vi "EnFlo_Tunnel_Display.vi"(4 "End Time":dbl, 5 "Start Time":dbl, 6 "Channel Values":dbl[](array[numeric]) format="%.3f", 7 "Ch names":string[](array[string])) -> ()   [LabVIEW 2016]
uses:
  Anemometry Sub Vis/Data_plotting_vis/File_Template_Clus.ctl
  Anemometry Sub Vis/Controls/Global_mode.ctl
  Anemometry Sub Vis/Globals/Constants_global.vi
  Anemometry Sub Vis/Data_plotting_vis/Results_plotter_Global.vi
  <vilib>/gmath/NI_Gmath.lvlib
panel:
  out "Inlet Door Heater Power %":dbl format="%#.2g"
  out "Exit Heater Power %":dbl format="%#.2g"
  out "Averaging time (minutes)":dbl format="%#.1f"
  out "End time":timestamp format="%<%H:%M\n%x>T"
  out "Start time":timestamp format="%<%H:%M\n%x>T"
  out "Top Level":bool
  out "Loop number":i32
  out "Lateral profiles":cluster{"Y Axis Current":dbl[], dbl[]}[](graph)
  out "Setpoints":dbl[](array[numeric])
  in  "Subtract Setpoint?":bool
  out "Vert Disp (mm)  @ 14m":dbl
  out "Inlet St Dev":dbl format="%#.3g"
  out "Inlet mapping":dbl[][](graph)=[[0.00729, 0.18153463174730816, 0.17352738437348433, 1.6752433719500537, 8.231465735195274, 17.570357598383207, 23.099772817121426, 25.58386930448374, 25.31727725753219, 24.28926231541072, 18.717383219374323, 10.355253339797807, 2.7760273383248344, 0.3109897541921306, 0.08276881403435009, 0.06197], [0.04411, 0.1361526368018142, 0.04039202183336771, 1.5611636795339547, 8.176972694107874, 17.32000974741714, 24.257541358764026, 25.949153465972987, 26.01802540761648, 25.060373307424115, 18.284750328365213, 8.689831176707928, 2.642937641487066, 0.43219350072447926, -0.019957690739617468, 0.07351], [0.05478, 0.03446320268089581, 0.2086595806581808, 1.6919212249796047, 6.580368005180591, 14.333585185483123, 21.06810094963999, 23.709254571137723, 24.04768940379576, 21.01660820522005, 13.60443428327954, 6.2766496258038735, 1.7988963349022484, 0.2952877651784204, 0.05436788410934033, 0.1022], [0.04013, 0.06419557464541133, 0.2035068586120256, 1.3118741659450193, 4.7061387064566835, 9.009825946069038, 12.927700276268434, 17.003135081884164, 16.83885730812343, 12.902263313363814, 8.246161922417906, 4.035269404379355, 1.329605659745338, 0.24574055091433544, 0.012829784119986217, 0.08755], [0.04404, 0.022691144295571734, 0.19102098261858932, 0.8525411026079828, 2.2353542219792946, 3.966676465246214, 6.305347763088489, 8.17672908183636, 7.7348668140659, 5.703994479070454, 3.8329088824353237, 1.9256956625267279, 0.6611488869641811, 0.20508248283573002, 0.10119553469307395, 0.08441]]
  out "Upstream Floor":cluster{"Array":dbl[], dbl[]}[](graph)
  in  "Averaging time (mins)":dbl=0.5 format="%.2f"
  in  "History in Minutes":dbl
  out "Strat":cluster{dbl[], dbl[]}[](graph)
  out "Des Air Temp":dbl format="%#.2g"
  out "Heat Extraction kW":dbl format="%#.2g"
  out "Av Pre Inlet Temp":dbl format="%#.2g"
  out "Av Exit  Temp":dbl format="%#.2g"
  out "Exit Dem Temp":dbl format="%#.2g"
  out "Heat Exchanger Valve %":dbl format="%#.1f"
  out "Delta T":dbl format="%#.2g"
  out "Pump Speed %":dbl format="%#.0f"
  out "Meas Delta P":dbl format="%#.2g"
  out "Desired Delta P":dbl format="%#.2f"
  out "Return Pressure":dbl format="%#.2g"
  out "Supply Pressure":dbl format="%#.2g"
  out "Max Motor Temp":dbl format="%#.1g"
  out "% Speed Tweak":dbl format="%#.2g"
  out "Shaft RPM":dbl format="%#.2g"
  out "Tunnel Speed  m/s":dbl format="%.3g"
  out "Uni Chilled water Temp":dbl format="%#.2g"
  out "Mixing Valve %":dbl format="%#.1f"
  out "Dem Temp":dbl
  out "Return Temp":dbl format="%#.2g"
  out "Supply Temp":dbl format="%#.2g"
  out "Floor_Cooling:Enable":bool
  out "Chiller_Pump:Enable":bool
  out "Panel Temps":cluster{"Array":dbl[], dbl[]}[](graph)
  in  "Stop Button":bool
  out "Heaters Enabled":bool
  out "Inlet Heaters":cluster{"yi":dbl[], dbl[]}[](graph)
  # "Chiller Pump Information"
  # "Chilled Water"
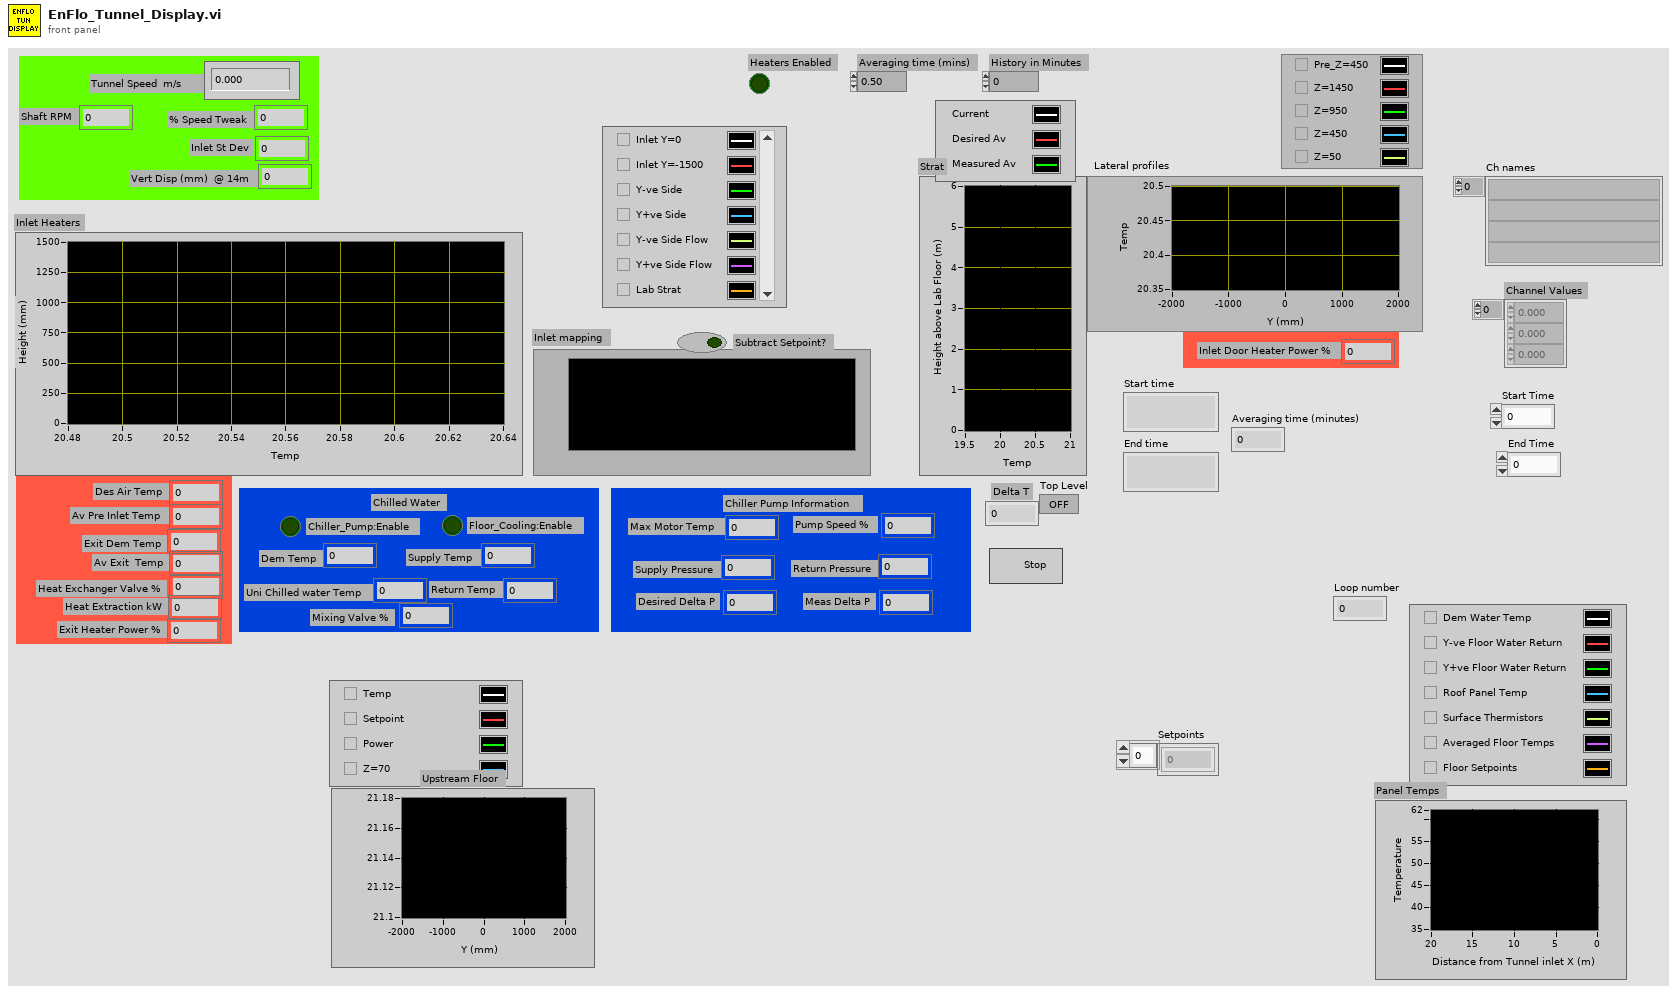
[diagram p1: front panel]
types:
  T1 = typedef "Global_mode.ctl" = enum16{"Read Global", "Load Global From File", "Write Global to File"}
  T2 = typedef "File_Template_Clus.ctl" = cluster{"Template Channel Name":string, "Description":string, "Tolerance":dbl, "Precision":string, "Folder level":string, "Source":string[], "Replace":string[], "Summarise":bool, "Dispose":bool, "Min Value":string, "Maths":string, "Omit Rows Containing":string[], "Ignore When":string[], "Max Value":string}
  T3 = cluster{"X Max":dbl, "Y Max ":dbl, "X Scale":cluster{"Xo":dbl, "delta X":dbl}, "Y Scale":cluster{"Xo":dbl, "delta X":dbl}, "X Values":dbl[], "Y Values":dbl[], "Z Max":dbl, "Z Min":dbl}
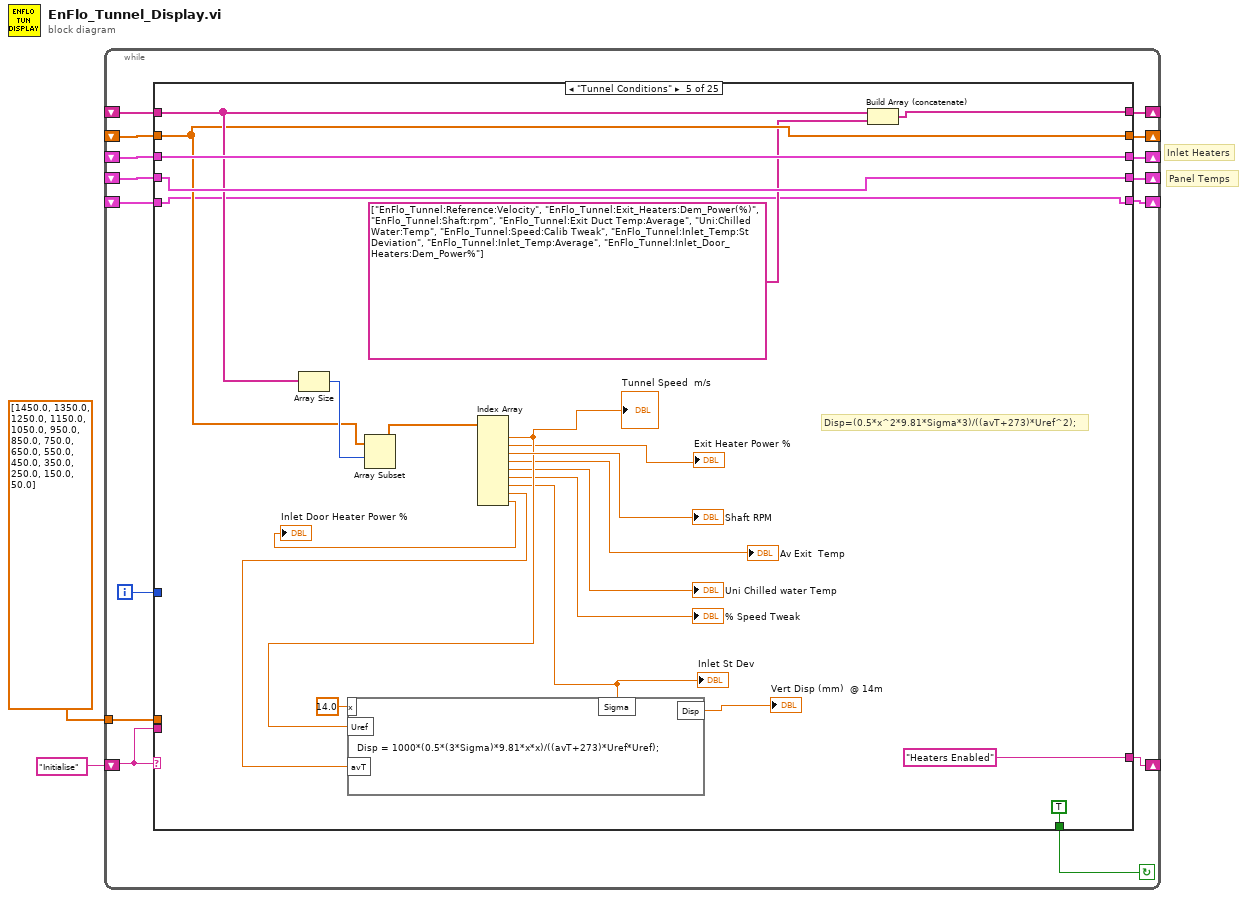
[diagram p0: block diagram]
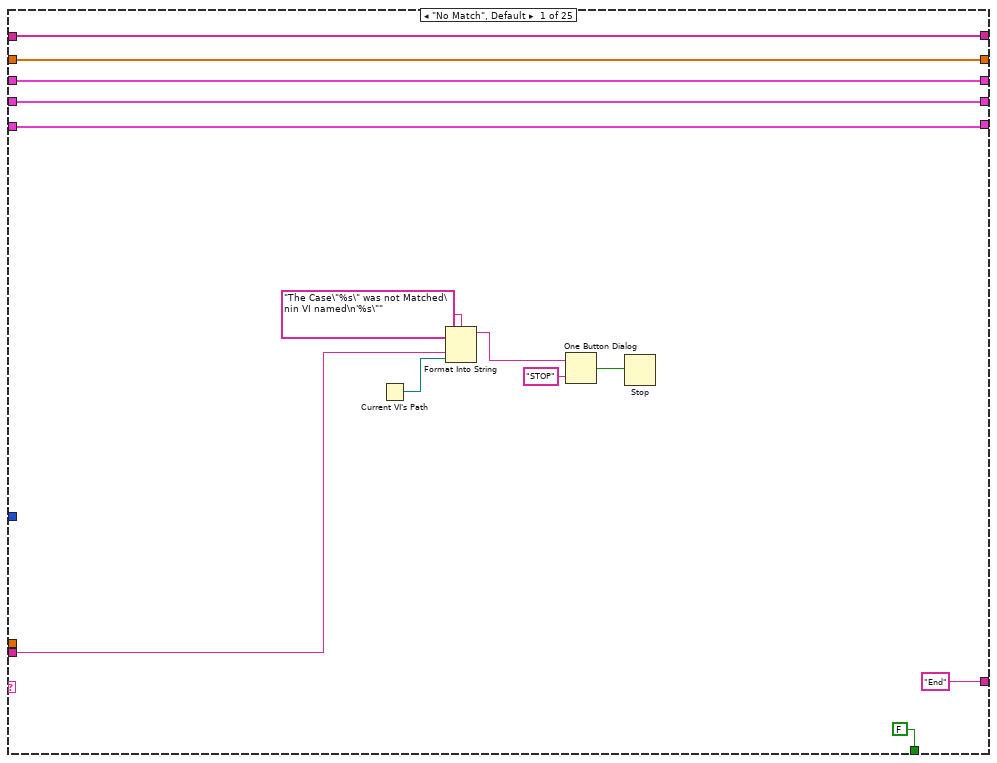
[diagram p2: hidden frame]
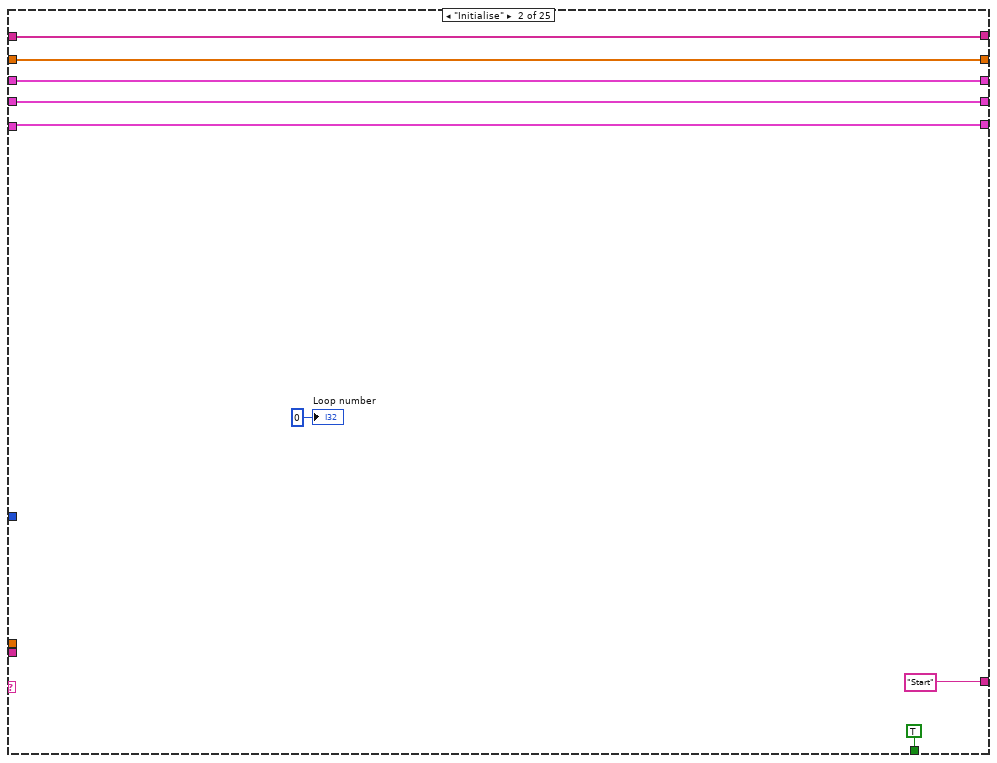
[diagram p3: hidden frame]
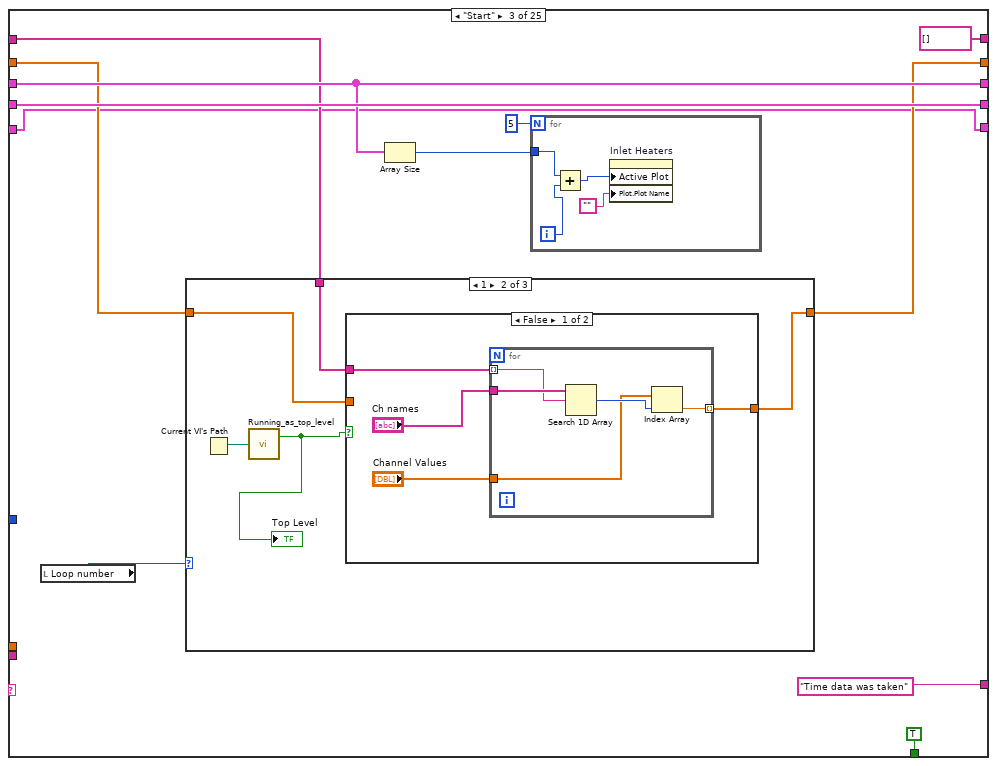
[diagram p4: hidden frame]
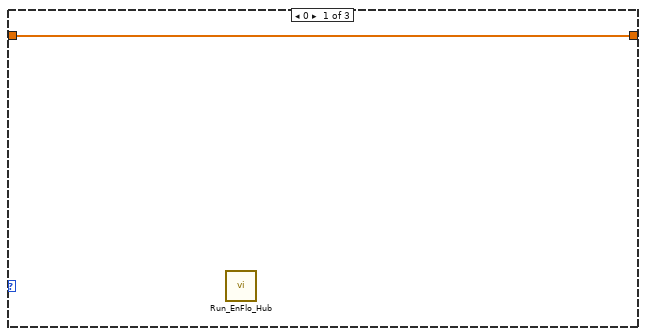
[diagram p5: hidden frame]
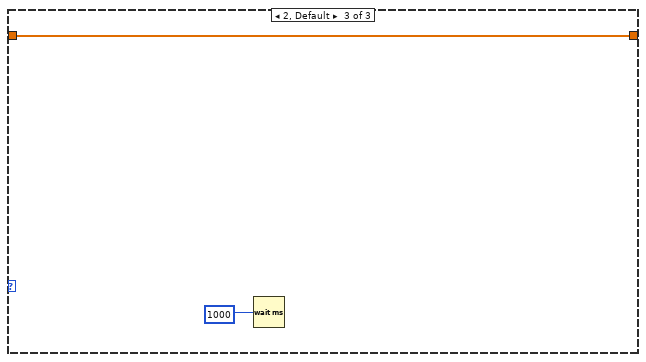
[diagram p7: hidden frame]
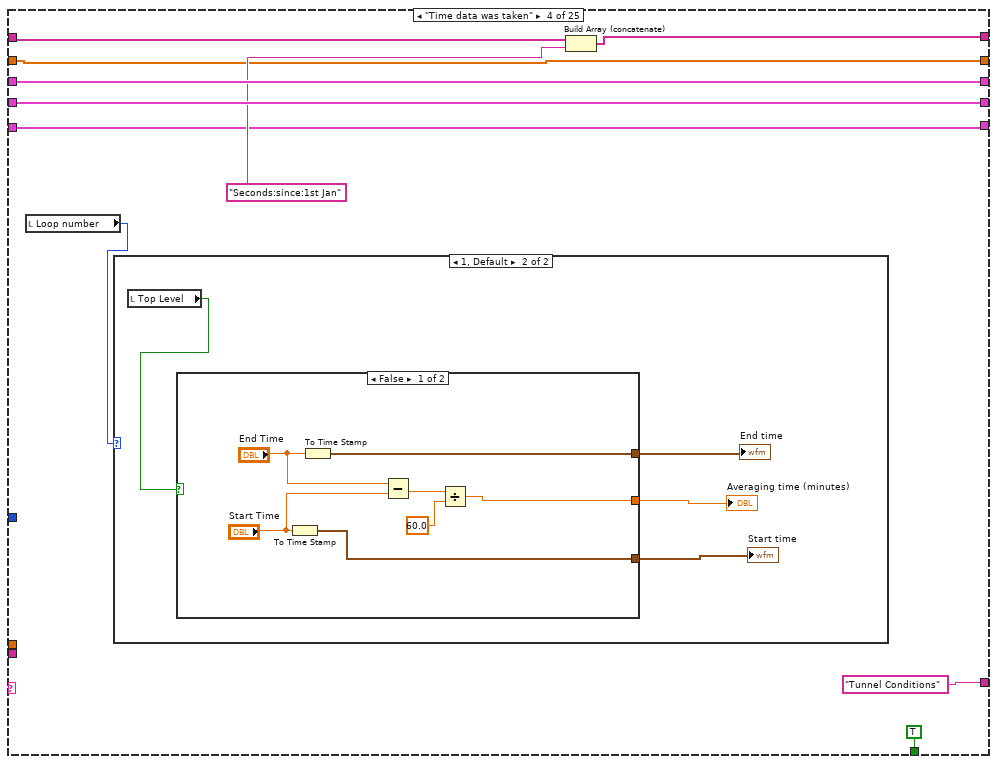
[diagram p8: hidden frame]
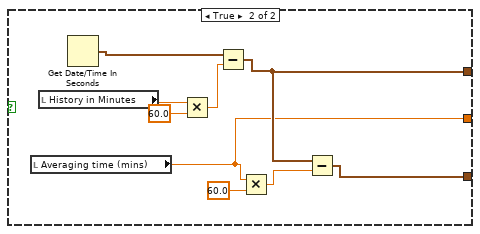
[diagram p10: hidden frame]
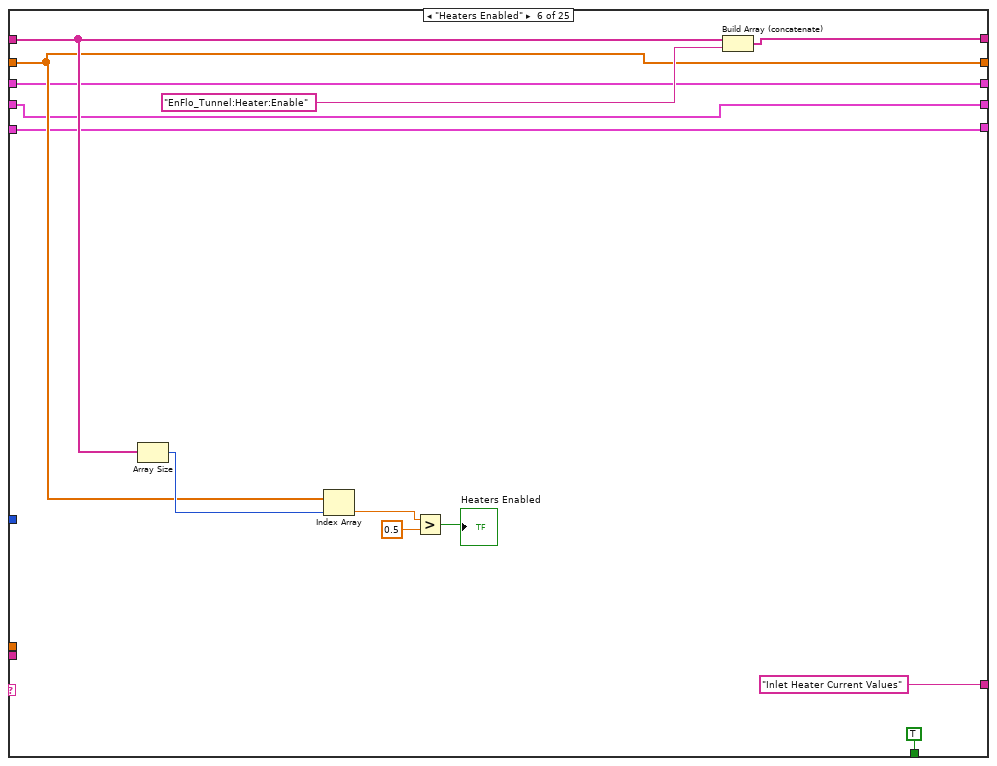
[diagram p11: hidden frame]
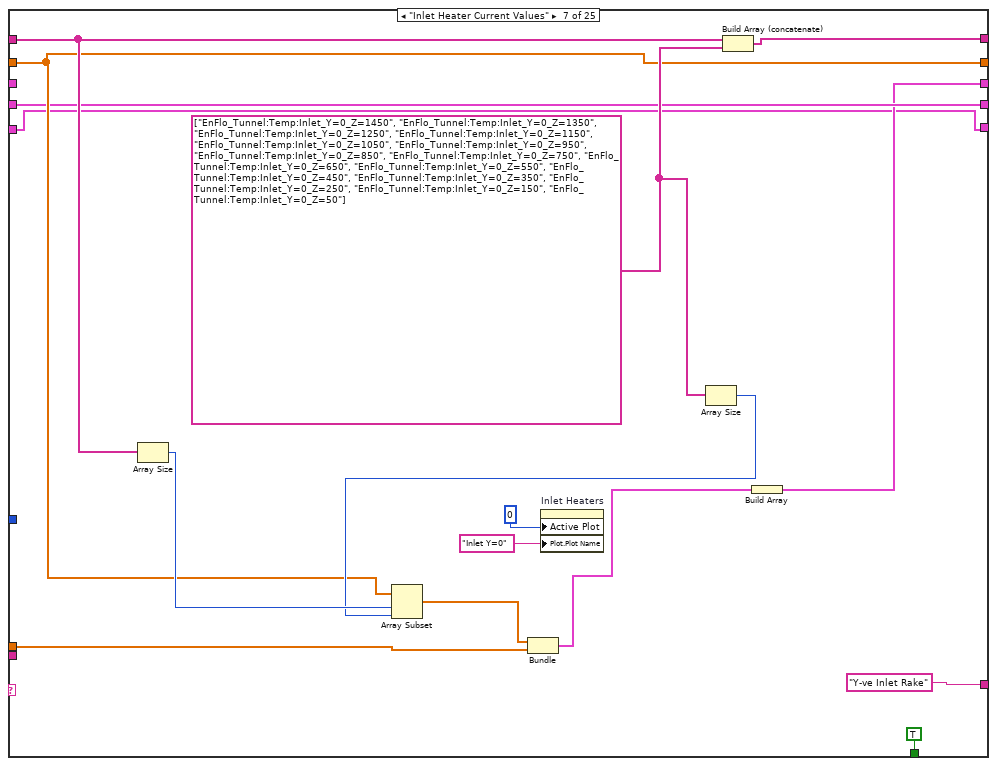
[diagram p12: hidden frame]
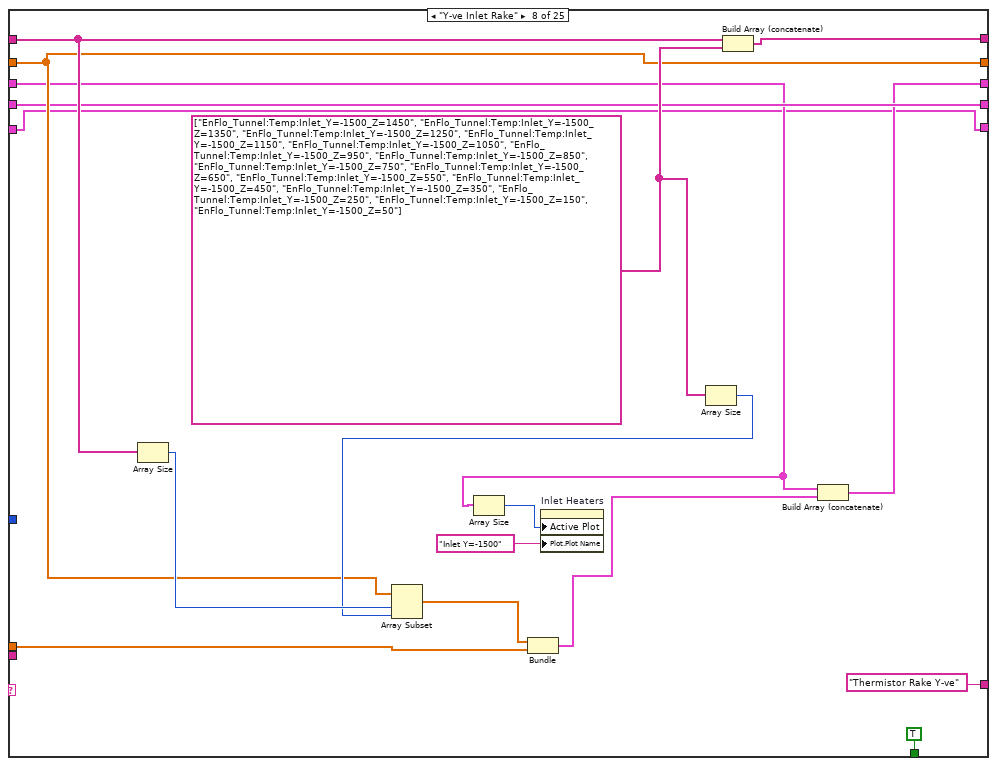
[diagram p13: hidden frame]
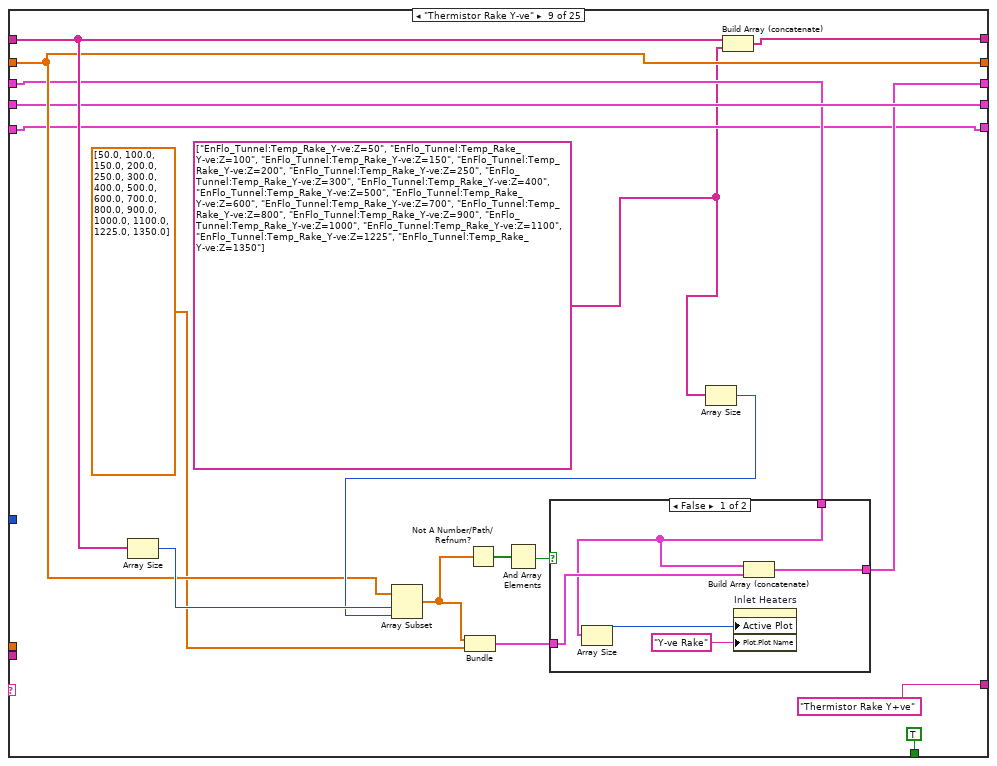
[diagram p14: hidden frame]
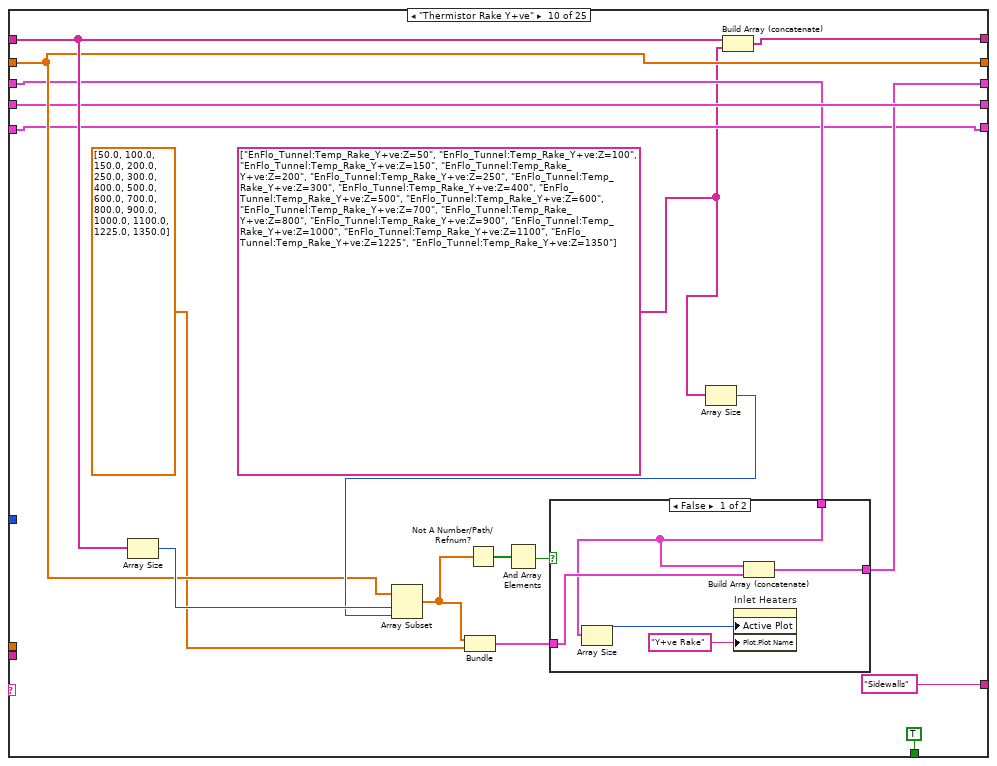
[diagram p16: hidden frame]
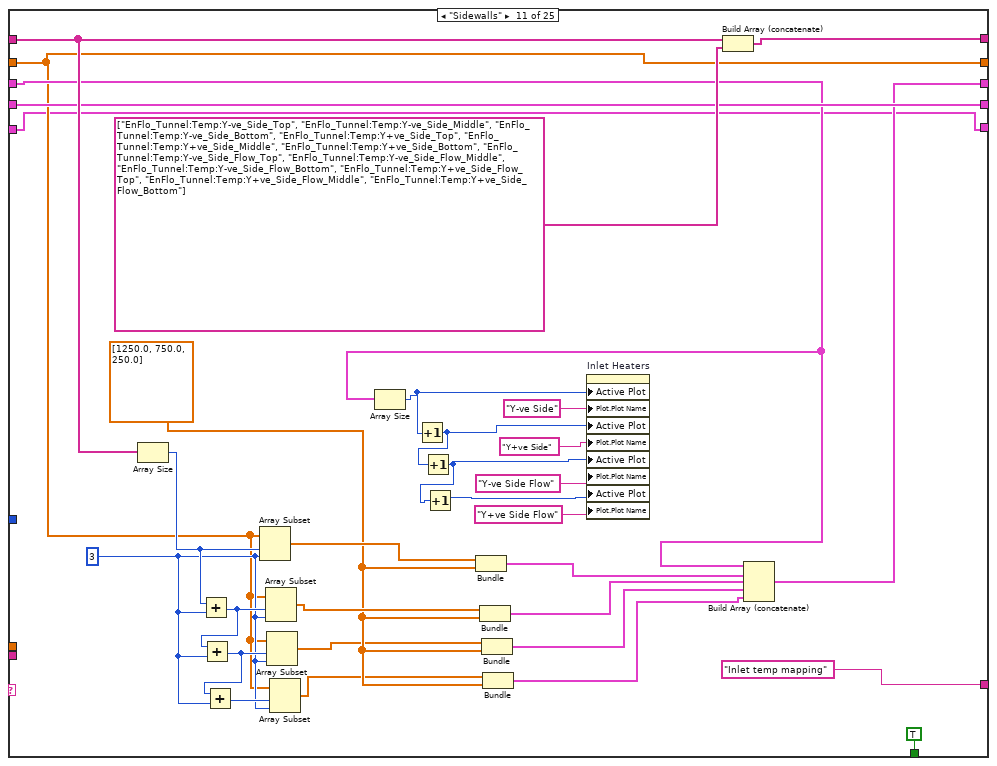
[diagram p18: hidden frame]
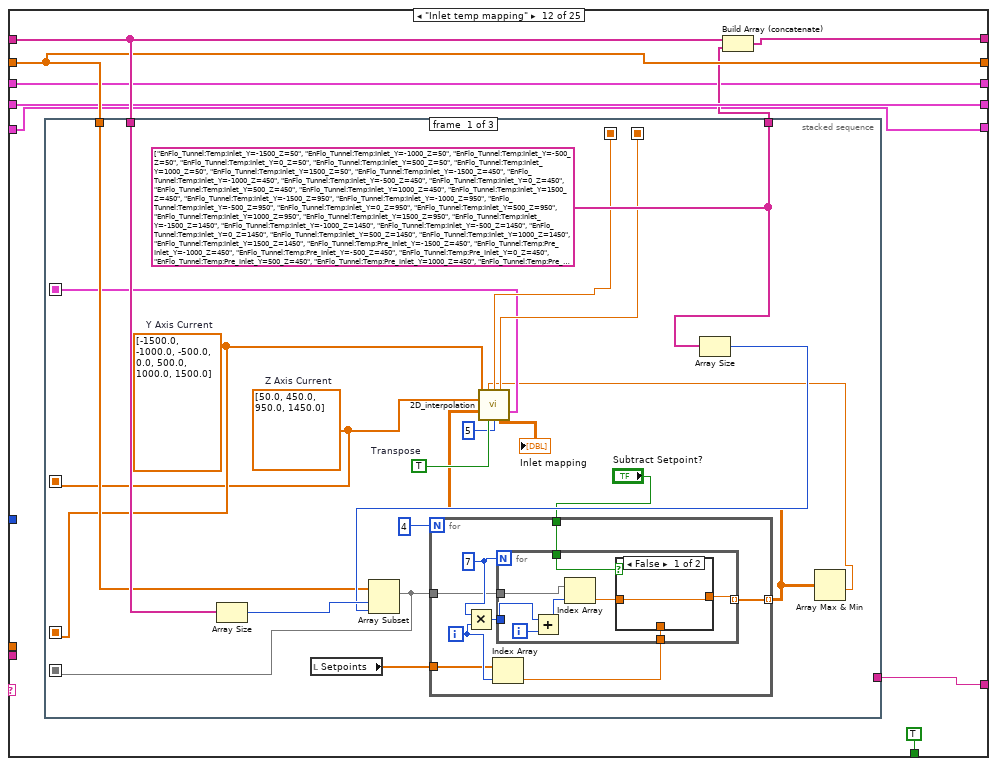
[diagram p19: hidden frame]
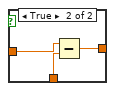
[diagram p20: hidden frame]
diagram:
  # "Panel Temps"
  # "Inlet Heaters"
  n1 = while {
    shift-right: [w15] -> _
    shift-left: "Initialise" -> [w16]
    shift-right: [w14] -> _
    shift-left: _ -> [w13]
    shift-right: [w11] -> _
    shift-left: _ -> [w12]
    shift-right: [w9] -> _
    shift-left: _ -> [w10]
    shift-right: [w8] -> _
    shift-left: _ -> [w7]
    tunnel: dbl[] [1450.0, 1350.0, 1250.0, 1150.0, 1050.0, 950.0, 850.0, 750.0, 650.0, 550.0, 450.0, 350.0, 250.0, 150.0, 50.0] -> [w5]
    shift-right: [w3] -> _
    shift-left: _ -> [w4]
    i -> [w6]
    stop <- w17 continue-if-true
    n2 = case shown="\"Tunnel Conditions\"" w16 {
      tunnel: [FALSE TRUE ("Top Level") TRUE TRUE ("Top Level") TRUE TRUE TRUE TRUE TRUE TRUE TRUE TRUE TRUE TRUE TRUE TRUE TRUE TRUE TRUE TRUE TRUE TRUE TRUE TRUE w591] -> w17
      tunnel: w16 -> [w24 _ _ _ _ _ _ _ _ _ _ _ _ _ _ _ _ _ _ _ _ _ _ _ _]
      tunnel: ["End" "Start" "Time data was taken" "Tunnel Conditions" "Heaters Enabled" "Inlet Heater Current Values" "Y-ve Inlet Rake" "Thermistor Rake Y-ve" "Thermistor Rake Y+ve" "Sidewalls" "Inlet temp mapping" w250 "EnFlo_Tunnel Chilled Water info" "EnFlo_Tunnel:Floor_Cooling:Enable" "Floor Panels Return Temps" "Roof Panel Values" "Upstream Floor Panel Temps" "Upstream Floor Panel Setpoints" "Upstream Floor Panel Powers" "Upstream Above Floor Panel" "Lab Stratification" w502 "Inlet Heater Power Values" "Get Server Values" "Start"] -> w15
      tunnel: [w22 w34 string[] [] w79 w122 w135 w151 w168 w186 w209 w246 w256 w337 w364 w377 w400 w430 w446 w463 w480 w497 w535 w562 w582 w588] -> w14
      tunnel: w13 -> [w22 w34 w41 w78 w117 w134 w150 w167 w185 w208 w245 w255 w336 w363 w376 w399 w429 w445 w462 w479 w496 w534 w561 w581 w588]
      tunnel: w12 -> [w21 w35 w42 w75 w116 w131 w147 w164 w182 w205 w220 w254 w333 w358 w373 w396 w426 w442 w459 w476 w493 w521 w558 w578 _]
      tunnel: [w21 w35 w43 w75 w116 w131 w147 w164 w182 w205 w220 w254 w333 w358 w373 w396 w426 w442 w459 w476 w493 w521 w558 w578 w590] -> w11
      tunnel: w10 -> [w20 w38 w47 w82 w121 w130 _ w156 w178 w201 w235 w251 w332 w362 w372 w394 w425 w441 w458 w475 w492 w504 w549 w570 w586]
      tunnel: [w20 w38 w47 w82 w121 w130 w140 w159 w179 w202 w241 w251 w332 w362 w372 w394 w425 w441 w458 w475 w492 w525 w556 w574 w586] -> w9
      tunnel: w7 -> [w19 w37 w48 w81 w120 w126 w146 w163 w181 w204 w244 w253 w328 w361 w368 _ w424 w437 w454 w471 w488 w533 w555 w576 w587]
      tunnel: [w19 w37 w48 w81 w120 w126 w146 w163 w181 w204 w244 w253 w328 w361 w368 w381 w423 w437 w454 w471 w488 w533 w555 w576 w587] -> w8
      tunnel: w6 -> [_ _ _ _ _ _ _ _ _ _ _ _ _ _ _ _ _ _ _ _ _ _ _ _ _]
      tunnel: w5 -> [_ _ _ _ _ _ w144 w161 _ _ _ _ _ _ _ _ _ _ _ _ _ w507 w550 w575 _]
      tunnel: w4 -> [w18 w31 w39 w73 w110 w125 w138 w154 w173 w196 w217 w249 w326 w339 w366 w379 w418 _ w451 w468 w485 w500 w545 w567 w584]
      tunnel: [w18 w31 w39 w73 w110 w125 w138 w154 w173 w196 w217 w249 w326 w339 w366 w379 w418 w435 w452 w469 w486 w500 w545 w567 w584] -> w3
      frame "No Match", Default {
        n3 = Current VI's Path() -> (path=w29:path)
        n4 = Format Into String(format string="The Case\"%s\" was not Matched\nin VI named\n'%s\"" ("Format String"), w24, w29) -> (resulting string=w26:string)  [unwired: 2 in, 1 out]
        n5 = One Button Dialog(message=w26, button name ("OK")="STOP") -> (true=w28:bool)
        n6 = Stop(stop? (T)=w28) -> ()
      }
      frame "Initialise" {
        "Loop number" <- 0 ("Loop number")
      }
      frame "Start" {
        n7 = local read "Loop number"() -> (w44:i32)
        n8 = case shown="1" w44 {
          tunnel: [w55 w59 w71] -> w43
          tunnel: w42 -> [w55 w57 w71]
          tunnel: w41 -> [_ w60 _]
          frame 0 {
            n9 = call "Run_EnFlo_Hub.vi"() -> ()  [unwired: 7 in, 1 out]
          }
          frame 1 {
            n10 = Current VI's Path() -> (path=w58:path)
            n11 = call "Running_as_top_level.vi"("Vi path name"=w58) -> ("Top Level"=w56:bool)  [unwired: 1 out]
            "Top Level" <- w56
            n12 = case shown="False" w56 {
              tunnel: w60 -> [w63 _]
              tunnel: [w61 w70] -> w59
              tunnel: w57 -> [_ w70]
              frame False {
                n13 = for {
                  tunnel: "Ch names" -> [w69]
                  tunnel: w63 -> [w68] mode=indexing
                  tunnel: "Channel Values" -> [w66]
                  tunnel: [w65] -> w61 mode=indexing
                  n14 = Search 1D Array(1D array=w69, element=w68) -> (index of element=w67:i32)  [unwired: 1 in]
                  n15 = Index Array(array=w66, index=w67) -> (element=w65:dbl)
                }
              }
              frame True {
              }
            }
          }
          frame 2, Default {
            n16 = Wait (ms)(milliseconds to wait=u32 1000 ("millisecond timer value")) -> ()  [unwired: 1 out]
          }
        }
        n17 = Array Size(array=w47) -> (size(s)=w45:i32)
        n18 = for {
          N: 5 -> [_]
          tunnel: w45 -> [w54]
          i -> [w53]
          n19 = Add(x=w54, y=w53) -> (x+y=w52:i32)
          n20 = property on="Inlet Heaters" class="XYGraph (strict)"("Active Plot"=w52, "Plot.Plot Name"="") -> ()  [unwired: 2 in, 2 out]
        }
      }
      frame "Time data was taken" {
        n21 = local read "Loop number"() -> (w74:i32)
        n22 = case shown="1, Default" w74 {
          frame 0 {
          }
          frame 1, Default {
            n23 = local read "Top Level"() -> (w84:bool)
            n24 = case shown="False" w84 {
              tunnel: [w93 w100] -> w86
              tunnel: [w92 w101] -> w85
              tunnel: [w87 w94] -> w83
              frame False {
                n25 = To Time Stamp(1:"Start Time") -> (0:w93:timestamp)
                n26 = To Time Stamp(1:"End Time") -> (0:w92:timestamp)
                n27 = Subtract(x="End Time", y="Start Time") -> (x-y=w89:dbl)
                n28 = Divide(x=w89, y=60.0) -> (x/y=w87:dbl)
              }
              frame True {
                n29 = local read "Averaging time (mins)"() -> (w94:dbl)
                n30 = local read "History in Minutes"() -> (w99:dbl)
                n31 = Get Date/Time In Seconds() -> (seconds since 1Jan1904=w102:timestamp)
                n32 = Multiply(x=w99, y=60.0) -> (x*y=w97:dbl)
                n33 = Subtract(x=w102, y=w97) -> (x-y=w101:timestamp)
                n34 = Multiply(x=w94, y=60.0) -> (x*y=w95:dbl)
                n35 = Subtract(x=w101, y=w95) -> (x-y=w100:timestamp)
              }
            }
            "Start time" <- w86
            "End time" <- w85
            "Averaging time (minutes)" <- w83
          }
        }
        n36 = Build Array (concatenate)(w78, "Seconds:since:1st Jan") -> (w79:string[])
      }
      frame "Tunnel Conditions" {
        # "Disp=(0.5*x^2*9.81*Sigma*3)/((avT+273)*Uref^2);"
        n37 = Array Size(array=w117) -> (size(s)=w119:i32)
        n38 = Array Subset(array=w116, index=w119) -> (w118:dbl[])  [unwired: 1 in]
        n39 = Index Array(array=w118) -> (element #1=w112:dbl, element #2=→"Exit Heater Power %":dbl, element #3=→"Shaft RPM":dbl, element #4=→"Av Exit  Temp":dbl, element #5=→"Uni Chilled water Temp":dbl, element #6=→"% Speed Tweak":dbl, element #7=w105:dbl, element #8=w104:dbl, element #9=→"Inlet Door Heater Power %":dbl)  [unwired: 9 in]
        "Tunnel Speed  m/s" <- w112
        "Inlet St Dev" <- w105
        n40 = formula code="Disp = 1000*(0.5*(3*Sigma)*9.81*x*x)/((avT+273)*Uref*Uref);"("x"=14.0 ("input variable"), "Uref"=w112, "Sigma"=w105, "avT"=w104) -> ("Disp"=→"Vert Disp (mm)  @ 14m":dbl)
        n41 = Build Array (concatenate)(w117, string[] ["EnFlo_Tunnel:Reference:Velocity", "EnFlo_Tunnel:Exit_Heaters:Dem_Power(%)", "EnFlo_Tunnel:Shaft:rpm", "EnFlo_Tunnel:Exit Duct Temp:Average", "Uni:Chilled Water:Temp", "EnFlo_Tunnel:Speed:Calib Tweak", "EnFlo_Tunnel:Inlet_Temp:St Deviation", "EnFlo_Tunnel:Inlet_Temp:Average", "EnFlo_Tunnel:Inlet_Door_Heaters:Dem_Power%"] ("subarray")) -> (w122:string[])
      }
      frame "Heaters Enabled" {
        n42 = Array Size(array=w134) -> (size(s)=w132:i32)
        n43 = Index Array(array=w131, index=w132) -> (element=w129:dbl)
        n44 = Greater?(x=w129, y=0.5) -> (0:→"Heaters Enabled":bool)
        n45 = Build Array (concatenate)(w134, "EnFlo_Tunnel:Heater:Enable" ("Ch Name")) -> (w135:string[])
      }
      frame "Inlet Heater Current Values" {
        w152 = string[] ["EnFlo_Tunnel:Temp:Inlet_Y=0_Z=1450", "EnFlo_Tunnel:Temp:Inlet_Y=0_Z=1350", "EnFlo_Tunnel:Temp:Inlet_Y=0_Z=1250", "EnFlo_Tunnel:Temp:Inlet_Y=0_Z=1150", "EnFlo_Tunnel:Temp:Inlet_Y=0_Z=1050", "EnFlo_Tunnel:Temp:Inlet_Y=0_Z=950", "EnFlo_Tunnel:Temp:Inlet_Y=0_Z=850", "EnFlo_Tunnel:Temp:Inlet_Y=0_Z=750", "EnFlo_Tunnel:Temp:Inlet_Y=0_Z=650", "EnFlo_Tunnel:Temp:Inlet_Y=0_Z=550", "EnFlo_Tunnel:Temp:Inlet_Y=0_Z=450", "EnFlo_Tunnel:Temp:Inlet_Y=0_Z=350", "EnFlo_Tunnel:Temp:Inlet_Y=0_Z=250", "EnFlo_Tunnel:Temp:Inlet_Y=0_Z=150", "EnFlo_Tunnel:Temp:Inlet_Y=0_Z=50"] ("subarray")
        n46 = Array Size(array=w150) -> (size(s)=w149:i32)
        n47 = property on="Inlet Heaters" class="XYGraph (strict)"("Active Plot"=u32 0, "Plot.Plot Name"="Inlet Y=0") -> ()  [unwired: 2 in, 2 out]
        n48 = Array Size(array=w152) -> (size(s)=w148:i32)
        n49 = Array Subset(array=w147, index=w149, length=w148) -> (w145:dbl[])
        n50 = Bundle(w145, w144) -> (w141:cluster{dbl[], dbl[]})  [unwired: 1 in]
        n51 = Build Array (concatenate)(w150, w152) -> (w151:string[])
        n52 = Build Array(w141) -> (w140:cluster{dbl[], dbl[]}[])
      }
      frame "Y-ve Inlet Rake" {
        w169 = string[] ["EnFlo_Tunnel:Temp:Inlet_Y=-1500_Z=1450", "EnFlo_Tunnel:Temp:Inlet_Y=-1500_Z=1350", "EnFlo_Tunnel:Temp:Inlet_Y=-1500_Z=1250", "EnFlo_Tunnel:Temp:Inlet_Y=-1500_Z=1150", "EnFlo_Tunnel:Temp:Inlet_Y=-1500_Z=1050", "EnFlo_Tunnel:Temp:Inlet_Y=-1500_Z=950", "EnFlo_Tunnel:Temp:Inlet_Y=-1500_Z=850", "EnFlo_Tunnel:Temp:Inlet_Y=-1500_Z=750", "EnFlo_Tunnel:Temp:Inlet_Y=-1500_Z=650", "EnFlo_Tunnel:Temp:Inlet_Y=-1500_Z=550", "EnFlo_Tunnel:Temp:Inlet_Y=-1500_Z=450", "EnFlo_Tunnel:Temp:Inlet_Y=-1500_Z=350", "EnFlo_Tunnel:Temp:Inlet_Y=-1500_Z=250", "EnFlo_Tunnel:Temp:Inlet_Y=-1500_Z=150", "EnFlo_Tunnel:Temp:Inlet_Y=-1500_Z=50"] ("subarray")
        n53 = Array Size(array=w167) -> (size(s)=w166:i32)
        n54 = Array Size(array=w156) -> (size(s)=w155:i32)
        n55 = property on="Inlet Heaters" class="XYGraph (strict)"("Active Plot"=w155, "Plot.Plot Name"="Inlet Y=-1500") -> ()  [unwired: 2 in, 2 out]
        n56 = Array Size(array=w169) -> (size(s)=w165:i32)
        n57 = Array Subset(array=w164, index=w166, length=w165) -> (w162:dbl[])
        n58 = Bundle(w162, w161) -> (w157:cluster{dbl[], dbl[]})  [unwired: 1 in]
        n59 = Build Array (concatenate)(w167, w169) -> (w168:string[])
        n60 = Build Array (concatenate)(w156, w157) -> (w159:cluster{"yi":dbl[], dbl[]}[])
      }
      frame "Thermistor Rake Y-ve" {
        w172 = string[] ["EnFlo_Tunnel:Temp_Rake_Y-ve:Z=50", "EnFlo_Tunnel:Temp_Rake_Y-ve:Z=100", "EnFlo_Tunnel:Temp_Rake_Y-ve:Z=150", "EnFlo_Tunnel:Temp_Rake_Y-ve:Z=200", "EnFlo_Tunnel:Temp_Rake_Y-ve:Z=250", "EnFlo_Tunnel:Temp_Rake_Y-ve:Z=300", "EnFlo_Tunnel:Temp_Rake_Y-ve:Z=400", "EnFlo_Tunnel:Temp_Rake_Y-ve:Z=500", "EnFlo_Tunnel:Temp_Rake_Y-ve:Z=600", "EnFlo_Tunnel:Temp_Rake_Y-ve:Z=700", "EnFlo_Tunnel:Temp_Rake_Y-ve:Z=800", "EnFlo_Tunnel:Temp_Rake_Y-ve:Z=900", "EnFlo_Tunnel:Temp_Rake_Y-ve:Z=1000", "EnFlo_Tunnel:Temp_Rake_Y-ve:Z=1100", "EnFlo_Tunnel:Temp_Rake_Y-ve:Z=1225", "EnFlo_Tunnel:Temp_Rake_Y-ve:Z=1350"] ("Sub set")
        n61 = Array Size(array=w185) -> (size(s)=w184:i32)
        n62 = Array Size(array=w172) -> (size(s)=w183:i32)
        n63 = Array Subset(array=w182, index=w184, length=w183) -> (w177:dbl[])
        n64 = Bundle(w177, dbl[] [50.0, 100.0, 150.0, 200.0, 250.0, 300.0, 400.0, 500.0, 600.0, 700.0, 800.0, 900.0, 1000.0, 1100.0, 1225.0, 1350.0]) -> (w174:cluster{dbl[], dbl[]})  [unwired: 1 in]
        n65 = Not A Number/Path/Refnum?(number/path/refnum=w177) -> (NaN/Path/Refnum?=w176:bool[])
        n66 = And Array Elements(Boolean array=w176) -> (logical AND=w175:bool)
        n67 = case shown="False" w175 {
          tunnel: [w192 w193] -> w179
          tunnel: w178 -> [w188 w193]
          tunnel: w174 -> [w191 _]
          frame False {
            n68 = Array Size(array=w188) -> (size(s)=w189:i32)
            n69 = property on="Inlet Heaters" class="XYGraph (strict)"("Active Plot"=w189, "Plot.Plot Name"="Y-ve Rake") -> ()  [unwired: 2 in, 2 out]
            n70 = Build Array (concatenate)(w188, w191) -> (w192:cluster{"yi":dbl[], dbl[]}[])
          }
          frame True {
          }
        }
        n71 = Build Array (concatenate)(w185, w172) -> (w186:string[])
      }
      frame "Thermistor Rake Y+ve" {
        w194 = string[] ["EnFlo_Tunnel:Temp_Rake_Y+ve:Z=50", "EnFlo_Tunnel:Temp_Rake_Y+ve:Z=100", "EnFlo_Tunnel:Temp_Rake_Y+ve:Z=150", "EnFlo_Tunnel:Temp_Rake_Y+ve:Z=200", "EnFlo_Tunnel:Temp_Rake_Y+ve:Z=250", "EnFlo_Tunnel:Temp_Rake_Y+ve:Z=300", "EnFlo_Tunnel:Temp_Rake_Y+ve:Z=400", "EnFlo_Tunnel:Temp_Rake_Y+ve:Z=500", "EnFlo_Tunnel:Temp_Rake_Y+ve:Z=600", "EnFlo_Tunnel:Temp_Rake_Y+ve:Z=700", "EnFlo_Tunnel:Temp_Rake_Y+ve:Z=800", "EnFlo_Tunnel:Temp_Rake_Y+ve:Z=900", "EnFlo_Tunnel:Temp_Rake_Y+ve:Z=1000", "EnFlo_Tunnel:Temp_Rake_Y+ve:Z=1100", "EnFlo_Tunnel:Temp_Rake_Y+ve:Z=1225", "EnFlo_Tunnel:Temp_Rake_Y+ve:Z=1350"] ("Sub set")
        n72 = Array Size(array=w208) -> (size(s)=w207:i32)
        n73 = Array Size(array=w194) -> (size(s)=w206:i32)
        n74 = Array Subset(array=w205, index=w207, length=w206) -> (w200:dbl[])
        n75 = Bundle(w200, dbl[] [50.0, 100.0, 150.0, 200.0, 250.0, 300.0, 400.0, 500.0, 600.0, 700.0, 800.0, 900.0, 1000.0, 1100.0, 1225.0, 1350.0]) -> (w197:cluster{dbl[], dbl[]})  [unwired: 1 in]
        n76 = Not A Number/Path/Refnum?(number/path/refnum=w200) -> (NaN/Path/Refnum?=w199:bool[])
        n77 = And Array Elements(Boolean array=w199) -> (logical AND=w198:bool)
        n78 = case shown="False" w198 {
          tunnel: [w215 w216] -> w202
          tunnel: w201 -> [w211 w216]
          tunnel: w197 -> [w214 _]
          frame False {
            n79 = Array Size(array=w211) -> (size(s)=w212:i32)
            n80 = property on="Inlet Heaters" class="XYGraph (strict)"("Active Plot"=w212, "Plot.Plot Name"="Y+ve Rake") -> ()  [unwired: 2 in, 2 out]
            n81 = Build Array (concatenate)(w211, w214) -> (w215:cluster{"yi":dbl[], dbl[]}[])
          }
          frame True {
          }
        }
        n82 = Build Array (concatenate)(w208, w194) -> (w209:string[])
      }
      frame "Sidewalls" {
        w223 = dbl[] [1250.0, 750.0, 250.0]
        w224 = 3 ("length")
        n83 = Array Size(array=w245) -> (size(s)=w240:i32)
        n84 = Add(x=w240, y=w224) -> (x+y=w226:i32)
        n85 = Add(x=w226, y=w224) -> (x+y=w225:i32)
        n86 = Add(x=w225, y=w224) -> (x+y=w227:i32)
        n87 = Array Subset(array=w220, index=w240, length=w224) -> (w239:dbl[])
        n88 = Array Subset(array=w220, index=w226, length=w224) -> (w238:dbl[])
        n89 = Array Subset(array=w220, index=w225, length=w224) -> (w222:dbl[])
        n90 = Array Subset(array=w220, index=w227, length=w224) -> (w221:dbl[])
        n91 = Array Size(array=w235) -> (size(s)=w233:i32)
        n92 = Increment(x=w233) -> (x+1=w230:i32)
        n93 = Increment(x=w230) -> (x+1=w228:i32)
        n94 = Increment(x=w228) -> (x+1=w229:i32)
        n95 = Bundle(w239, w223) -> (w242:cluster{dbl[], dbl[]})  [unwired: 1 in]
        n96 = Bundle(w238, w223) -> (w237:cluster{dbl[], dbl[]})  [unwired: 1 in]
        n97 = Bundle(w222, w223) -> (w219:cluster{dbl[], dbl[]})  [unwired: 1 in]
        n98 = Bundle(w221, w223) -> (w218:cluster{dbl[], dbl[]})  [unwired: 1 in]
        n99 = property on="Inlet Heaters" class="XYGraph (strict)"("Active Plot"=w233, "Plot.Plot Name"="Y-ve Side", "Active Plot"=w230, "Plot.Plot Name"="Y+ve Side", "Active Plot"=w228, "Plot.Plot Name"="Y-ve Side Flow", "Active Plot"=w229, "Plot.Plot Name"="Y+ve Side Flow") -> ()  [unwired: 2 in, 2 out]
        n100 = Build Array (concatenate)(w245, string[] ["EnFlo_Tunnel:Temp:Y-ve_Side_Top", "EnFlo_Tunnel:Temp:Y-ve_Side_Middle", "EnFlo_Tunnel:Temp:Y-ve_Side_Bottom", "EnFlo_Tunnel:Temp:Y+ve_Side_Top", "EnFlo_Tunnel:Temp:Y+ve_Side_Middle", "EnFlo_Tunnel:Temp:Y+ve_Side_Bottom", "EnFlo_Tunnel:Temp:Y-ve_Side_Flow_Top", "EnFlo_Tunnel:Temp:Y-ve_Side_Flow_Middle", "EnFlo_Tunnel:Temp:Y-ve_Side_Flow_Bottom", "EnFlo_Tunnel:Temp:Y+ve_Side_Flow_Top", "EnFlo_Tunnel:Temp:Y+ve_Side_Flow_Middle", "EnFlo_Tunnel:Temp:Y+ve_Side_Flow_Bottom"] ("subarray")) -> (w246:string[])
        n101 = Build Array (concatenate)(w235, w242, w237, w219, w218) -> (w241:cluster{"yi":dbl[], dbl[]}[])
      }
      frame "Inlet temp mapping" {
        n102 = stacked-sequence {
          seq-local: [w268 _ _] -> [_ w305 _]
          seq-local: [w267 _ _] -> [_ w306 _]
          seq-local: [w266 _ _] -> [_ w301 _]
          seq-local: [w260 _ _] -> [_ _ w316]
          seq-local: [w259 _ _] -> [_ _ w317]
          seq-local: [w258 _ _] -> [_ _ _]
          tunnel: w255 -> [w276 _ _]
          tunnel: w254 -> [w273 _ _]
          tunnel: [w272 _ _] -> w252
          tunnel: [_ "EnFlo_Tunnel:Chiller_Pump:Enable" _] -> w250
          frame #0 {
            w270 = TRUE  # Transpose
            w258 = dbl[] [50.0, 450.0, 950.0, 1450.0]  # Z Axis Current
            w259 = dbl[] [-1500.0, -1000.0, -500.0, 0.0, 500.0, 1000.0, 1500.0]  # Y Axis Current
            w272 = string[] ["EnFlo_Tunnel:Temp:Inlet_Y=-1500_Z=50", "EnFlo_Tunnel:Temp:Inlet_Y=-1000_Z=50", "EnFlo_Tunnel:Temp:Inlet_Y=-500_Z=50", "EnFlo_Tunnel:Temp:Inlet_Y=0_Z=50", "EnFlo_Tunnel:Temp:Inlet_Y=500_Z=50", "EnFlo_Tunnel:Temp:Inlet_Y=1000_Z=50", "EnFlo_Tunnel:Temp:Inlet_Y=1500_Z=50", "EnFlo_Tunnel:Temp:Inlet_Y=-1500_Z=450", "EnFlo_Tunnel:Temp:Inlet_Y=-1000_Z=450", "EnFlo_Tunnel:Temp:Inlet_Y=-500_Z=450", "EnFlo_Tunnel:Temp:Inlet_Y=0_Z=450", "EnFlo_Tunnel:Temp:Inlet_Y=500_Z=450", "EnFlo_Tunnel:Temp:Inlet_Y=1000_Z=450", "EnFlo_Tunnel:Temp:Inlet_Y=1500_Z=450", "EnFlo_Tunnel:Temp:Inlet_Y=-1500_Z=950", "EnFlo_Tunnel:Temp:Inlet_Y=-1000_Z=950", "EnFlo_Tunnel:Temp:Inlet_Y=-500_Z=950", "EnFlo_Tunnel:Temp:Inlet_Y=0_Z=950", "EnFlo_Tunnel:Temp:Inlet_Y=500_Z=950", "EnFlo_Tunnel:Temp:Inlet_Y=1000_Z=950", "EnFlo_Tunnel:Temp:Inlet_Y=1500_Z=950", "EnFlo_Tunnel:Temp:Inlet_Y=-1500_Z=1450", "EnFlo_Tunnel:Temp:Inlet_Y=-1000_Z=1450", "EnFlo_Tunnel:Temp:Inlet_Y=-500_Z=1450", "EnFlo_Tunnel:Temp:Inlet_Y=0_Z=1450", "EnFlo_Tunnel:Temp:Inlet_Y=500_Z=1450", "EnFlo_Tunnel:Temp:Inlet_Y=1000_Z=1450", "EnFlo_Tunnel:Temp:Inlet_Y=1500_Z=1450", "EnFlo_Tunnel:Temp:Pre_Inlet_Y=-1500_Z=450", "EnFlo_Tunnel:Temp:Pre_Inlet_Y=-1000_Z=450", "EnFlo_Tunnel:Temp:Pre_Inlet_Y=-500_Z=450", "EnFlo_Tunnel:Temp:Pre_Inlet_Y=0_Z=450", "EnFlo_Tunnel:Temp:Pre_Inlet_Y=500_Z=450", "EnFlo_Tunnel:Temp:Pre_Inlet_Y=1000_Z=450", "EnFlo_Tunnel:Temp:Pre_Inlet_Y=1500_Z=450"] ("subarray")
            n103 = Array Size(array=w276) -> (size(s)=w275:i32)
            n104 = local read "Setpoints"() -> (w264:dbl[])
            n105 = Array Size(array=w272) -> (size(s)=w274:i32)
            n106 = Array Subset(array=w273, index=w275, length=w274) -> (w260:dbl[])
            n107 = for {
              N: 4 -> [_]
              tunnel: [w282] -> w262 mode=indexing
              tunnel: w264 -> [w280]
              tunnel: "Subtract Setpoint?" -> [w279]
              tunnel: w260 -> [w277]
              i -> [w281]
              w284 = 7
              n108 = Multiply(x=w284, y=w281) -> (x*y=w283:i32)
              n109 = Index Array(array=w280, index=w281) -> (element=w278:dbl)
              n110 = for {
                N: w284 -> [_]
                tunnel: w283 -> [w291]
                tunnel: w277 -> [w289]
                tunnel: [w285] -> w282 mode=indexing
                tunnel: w279 -> [w288]
                tunnel: w278 -> [w286]
                i -> [w292]
                n111 = Add(x=w291, y=w292) -> (x+y=w290:i32)
                n112 = Index Array(array=w289, index=w290) -> (element=w287:dbl)
                n113 = case shown="False" w288 {
                  tunnel: w287 -> [w293 w296]
                  tunnel: w286 -> [_ w295]
                  tunnel: [w293 w294] -> w285
                  frame False {
                  }
                  frame True {
                    n114 = Subtract(x=w296, y=w295) -> (x-y=w294:dbl)
                  }
                }
              }
            }
            n115 = Array Max & Min(array=w262) -> (min value=w261:dbl)  [unwired: 3 out]
            n116 = call "2D_interpolation.vi"("X Axis Current"=w259, "Min Z Value In"=w261, "Y axis Current"=w258, "Plot In"=w262, "Transpose"=w270, "Point Size"=5) -> ("min Z value"=w268:dbl, "max Z value"=w267:dbl, "Axis info"=w266:T3, "Plot Out"=→"Inlet mapping":dbl[][])  [unwired: 2 in, 4 out]
          }
          frame #1 {
            w302 = u8 0 ("X Scale.Display Format:Precision")
            n117 = Bundle("max Z value"=w306, u32 16721152) -> (w309:cluster{"max Z value":dbl, u32})  [unwired: 1 out]
            n118 = Bundle("min Z value"=w305, u32 3743) -> (w310:cluster{"min Z value":dbl, u32})  [unwired: 1 out]
            n119 = Unbundle By Name(w301) -> ("Y Scale"=w300:cluster{"Xo":dbl, "delta X":dbl}, "Y Max"=w299:dbl, "X Scale"=w298:cluster{"Xo":dbl, "delta X":dbl}, "X Max"=w297:dbl)
            n120 = Build Array(w309, w310) -> (w303:cluster{"min Z value":dbl, u32}[])
            n121 = property on="Inlet mapping" class="IntGraph (strict)"("Ignore Array"=FALSE, "ZScale.MarkerVals[]"=w303, "XScale.Ofst&Mult"=w300, "XScale.Maximum"=w299, "YScale.Ofst&Mult"=w298, "YScale.Maximum"=w297, "XScale.Precision"=w302, "YScale.Precision"=w302) -> ()  [unwired: 2 in, 2 out]
          }
          frame #2 {
            n122 = for {
              N: 5 -> [_]
              tunnel: w317 -> [w325]
              tunnel: w316 -> [w324]
              tunnel: [w319] -> w314 mode=indexing
              i -> [w321]
              w323 = 7 ("length")
              n123 = Multiply(x=w321, y=w323) -> (x*y=w322:i32)
              n124 = Array Subset(array=w324, index=w322, length=w323) -> (w320:dbl[])
              n125 = Bundle("Y Axis Current"=w325, w320) -> (w319:cluster{"Y Axis Current":dbl[], dbl[]})  [unwired: 1 in]
            }
            n126 = local read "Loop number"() -> (w312:i32)
            n127 = Reverse 1D Array(array=w314) -> (reversed array=w313:cluster{"Y Axis Current":dbl[], dbl[]}[])
            n128 = case shown="1, Default" w312 {
              tunnel: w313 -> [_ w318]
              frame 0 {
              }
              frame 1, Default {
                "Lateral profiles" <- w318
              }
            }
          }
        }
        n129 = Build Array (concatenate)(w255, w252) -> (w256:string[])
      }
      frame "EnFlo_Tunnel:Chiller_Pump:Enable" {
        n130 = Array Size(array=w336) -> (size(s)=w334:i32)
        n131 = Index Array(array=w333, index=w334) -> (element=w331:dbl)
        n132 = Greater?(x=w331, y=0.5) -> (0:→"Chiller_Pump:Enable":bool)
        n133 = Build Array (concatenate)(w336, "EnFlo_Tunnel:Chiller_Pump:Enable" ("Ch Name")) -> (w337:string[])
      }
      frame "EnFlo_Tunnel Chilled Water info" {
        n134 = Array Size(array=w363) -> (size(s)=w357:i32)
        n135 = Array Subset(array=w358, index=w357) -> (w356:dbl[])  [unwired: 1 in]
        n136 = Index Array(array=w356) -> (element #1=→"Supply Temp":dbl, element #2=→"Return Temp":dbl, element #3=→"Dem Temp":dbl, element #4=→"Mixing Valve %":dbl, element #5=w343:dbl, element #6=w342:dbl, element #7=→"Heat Exchanger Valve %":dbl, element #8=→"Exit Dem Temp":dbl, element #9=w348:dbl, element #10=w347:dbl, element #11=→"Desired Delta P":dbl, element #12=w340:dbl)  [unwired: 12 in]
        "Supply Pressure" <- w348
        "Return Pressure" <- w347
        n137 = Multiply(x=w340, y=10.0) -> (x*y=→"Pump Speed %":dbl)
        n138 = Max & Min(x=w343, y=w342) -> (max(x,y)=→"Max Motor Temp":dbl)  [unwired: 1 out]
        n139 = Build Array (concatenate)(w363, string[] ["EnFlo_Tunnel:Chilled Water:Supply", "EnFlo_Tunnel:Chilled Water:Return", "EnFlo_Tunnel:Chilled Water:Dem Temp", "EnFlo_Tunnel:Chilled Water:Valve Dem Pos", "EnFlo_Tunnel:Chilled Water:Motor1 Temp", "EnFlo_Tunnel:Chilled Water:Motor2 Temp", "EnFlo_Tunnel:Heat_Ex_Div_Valve:Dem Pos", "EnFlo_Tunnel:Exit Duct:Dem Temp", "EnFlo_Tunnel:Chilled Water:Pressure_supply (Bar)", "EnFlo_Tunnel:Chilled Water:Pressure_return (Bar)", "EnFlo_Tunnel:Chilled Water:Desired_Delta_P", "EnFlo_Tunnel:Chilled Water:Motor_Dem_Voltage"] ("subarray")) -> (w364:string[])
        n140 = Subtract(x=w348, y=w347) -> (x-y=→"Meas Delta P":dbl)
      }
      frame "EnFlo_Tunnel:Floor_Cooling:Enable" {
        n141 = Array Size(array=w376) -> (size(s)=w374:i32)
        n142 = Index Array(array=w373, index=w374) -> (element=w371:dbl)
        n143 = Greater?(x=w371, y=0.5) -> (0:→"Floor_Cooling:Enable":bool)
        n144 = Build Array (concatenate)(w376, "EnFlo_Tunnel:Floor_Cooling:Enable" ("Ch Name")) -> (w377:string[])
      }
      frame "Floor Panels Return Temps" {
        w393 = string[] ["EnFlo_Tunnel:Return_Temp:Floor_Far_02", "EnFlo_Tunnel:Return_Temp:Floor_Near_02", "EnFlo_Tunnel:Return_Temp:Floor_Far_03", "EnFlo_Tunnel:Return_Temp:Floor_Near_03", "EnFlo_Tunnel:Return_Temp:Floor_Far_04", "EnFlo_Tunnel:Return_Temp:Floor_Near_04", "EnFlo_Tunnel:Return_Temp:Floor_Far_05", "EnFlo_Tunnel:Return_Temp:Floor_Near_05", "EnFlo_Tunnel:Return_Temp:Floor_Far_06", "EnFlo_Tunnel:Return_Temp:Floor_Near_06", "EnFlo_Tunnel:Return_Temp:Floor_Far_07", "EnFlo_Tunnel:Return_Temp:Floor_Near_07", "EnFlo_Tunnel:Return_Temp:Floor_Far_08", "EnFlo_Tunnel:Return_Temp:Floor_Near_08", "EnFlo_Tunnel:Return_Temp:Floor_Far_09", "EnFlo_Tunnel:Return_Temp:Floor_Near_09", "EnFlo_Tunnel:Return_Temp:Floor_Far_10", "EnFlo_Tunnel:Return_Temp:Floor_Near_10", "EnFlo_Tunnel:Return_Temp:Floor_Far_11", "EnFlo_Tunnel:Return_Temp:Floor_Near_11", "EnFlo_Tunnel:Return_Temp:Floor_Far_12", "EnFlo_Tunnel:Return_Temp:Floor_Near_12", "EnFlo_Tunnel:Return_Temp:Floor_Far_13", "EnFlo_Tunnel:Return_Temp:Floor_Near_13", "EnFlo_Tunnel:Return_Temp:Floor_Far_14", "EnFlo_Tunnel:Return_Temp:Floor_Turn_14", "EnFlo_Tunnel:Return_Temp:Floor_Turn_Sur_14", "EnFlo_Tunnel:Return_Temp:Floor_Turn_Sur_15", "EnFlo_Tunnel:Return_Temp:Floor_Far_16", "EnFlo_Tunnel:Return_Temp:Floor_Near_16", "EnFlo_Tunnel:Return_Temp:Floor_Far_17", "EnFlo_Tunnel:Return_Temp:Floor_Near_17", "EnFlo_Tunnel:Return_Temp:Floor_Far_18", "EnFlo_Tunnel:Return_Temp:Floor_Near_18", "EnFlo_Tunnel:Return_Temp:Floor_Far_19", "EnFlo_Tunnel:Return_Temp:Floor_Near_19"] ("subarray")
        n145 = Array Size(array=w399) -> (size(s)=w398:i32)
        n146 = local read "Dem Temp"() -> (w387:dbl)
        n147 = for {
          N: 18 -> [_]
          tunnel: [w416] -> w388 mode=indexing
          tunnel: w387 -> [w414]
          tunnel: [w414] -> w386 mode=indexing
          i -> [w417]
          n148 = Add(x=1.5, y=w417) -> (x+y=w416:dbl)
        }
        n149 = Bundle(w388, w386) -> (w382:cluster{dbl[], dbl[]})  [unwired: 1 in]
        n150 = Array Size(array=w393) -> (size(s)=w397:i32)
        n151 = Array Subset(array=w396, index=w398, length=w397) -> (w392:dbl[])
        n152 = Decimate 1D Array(w392) -> (w383:dbl[], w391:dbl[])
        n153 = Not A Number/Path/Refnum?(number/path/refnum=w383) -> (NaN/Path/Refnum?=w385:bool[])
        n154 = And Array Elements(Boolean array=w385) -> (logical AND=w384:bool)
        n155 = Bundle(w388, w383) -> (w390:cluster{dbl[], dbl[]})  [unwired: 1 in]
        n156 = Bundle(w388, w391) -> (w389:cluster{dbl[], dbl[]})  [unwired: 1 in]
        n157 = Build Array(w390, w389, w382) -> (w380:cluster{dbl[], dbl[]}[])
        n158 = case shown="True" w384 {
          tunnel: w382 -> [_ w413]
          tunnel: [w408 w412] -> w381
          tunnel: w380 -> [w408 _]
          frame False {
            n159 = property on="Panel Temps" class="XYGraph (strict)"("Active Plot"=u32 0, "Plot.Plot Name"="Dem Water Temp", "Active Plot"=u32 1, "Plot.Plot Name"="Y-ve Floor Water Return", "Active Plot"=u32 2, "Plot.Plot Name"="Y+ve Floor Water Return") -> ()  [unwired: 2 in, 2 out]
          }
          frame True {
            n160 = property on="Panel Temps" class="XYGraph (strict)"("Active Plot"=u32 0, "Plot.Plot Name"="Dem Water Temp") -> ()  [unwired: 2 in, 2 out]
            n161 = Build Array(w413) -> (w412:cluster{dbl[], dbl[]}[])
          }
        }
        n162 = Build Array (concatenate)(w399, w393) -> (w400:string[])
      }
      frame "Roof Panel Values" {
        w421 = string[] ["EnFlo_Tunnel:Temp:Roof_Far_2", "EnFlo_Tunnel:Temp:Roof_Near_3", "EnFlo_Tunnel:Temp:Roof_Far_4", "EnFlo_Tunnel:Temp:Roof_Far_6", "EnFlo_Tunnel:Temp:Roof_Near_7", "EnFlo_Tunnel:Temp:Roof_Far_8", "EnFlo_Tunnel:Temp:Roof_Far_10", "EnFlo_Tunnel:Temp:Roof_Near_12", "EnFlo_Tunnel:Temp:Roof_Far_15", "EnFlo_Tunnel:Temp:Roof_Far_19"] ("subarray")
        n163 = Array Size(array=w429) -> (size(s)=w428:i32)
        n164 = Array Size(array=w421) -> (size(s)=w427:i32)
        n165 = Array Subset(array=w426, index=w428, length=w427) -> (w422:dbl[])
        n166 = Build Array (concatenate)(w429, w421) -> (w430:string[])
        n167 = Bundle(dbl[] [1.5, 2.5, 3.5, 5.5, 6.5, 7.5, 9.5, 11.5, 14.5, 18.5], w422) -> (w419:cluster{dbl[], dbl[]})  [unwired: 1 in]
        n168 = Build Array (concatenate)(w424, w419) -> (w423:cluster{dbl[], dbl[]}[])
      }
      frame "Upstream Floor Panel Temps" {
        w438 = string[] ["EnFlo_Tunnel:Temp:Floor_Up_Y=-1585", "EnFlo_Tunnel:Temp:Floor_Up_Y=-1250", "EnFlo_Tunnel:Temp:Floor_Up_Y=-920", "EnFlo_Tunnel:Temp:Floor_Up_Y=-585", "EnFlo_Tunnel:Temp:Floor_Up_Y=-250", "EnFlo_Tunnel:Temp:Floor_Up_Y=80", "EnFlo_Tunnel:Temp:Floor_Up_Y=415", "EnFlo_Tunnel:Temp:Floor_Up_Y=750", "EnFlo_Tunnel:Temp:Floor_Up_Y=1080", "EnFlo_Tunnel:Temp:Floor_Up_Y=1415"] ("subarray")
        n169 = Array Size(array=w445) -> (size(s)=w444:i32)
        n170 = Array Size(array=w438) -> (size(s)=w443:i32)
        n171 = Array Subset(array=w442, index=w444, length=w443) -> (w440:dbl[])
        n172 = Build Array (concatenate)(w445, w438) -> (w446:string[])
        n173 = property on="Upstream Floor" class="XYGraph (strict)"("Active Plot"=u32 0, "Plot.Plot Name"="Temp") -> ()  [unwired: 2 in, 2 out]
        n174 = Bundle("Array"=dbl[] [-1585.0, -1250.0, -920.0, -585.0, -250.0, 80.0, 415.0, 750.0, 1080.0, 1415.0], w440) -> (w436:cluster{"Array":dbl[], dbl[]})  [unwired: 1 in]
        n175 = Build Array(w436) -> (w435:cluster{"Array":dbl[], dbl[]}[])
      }
      frame "Upstream Floor Panel Setpoints" {
        w455 = string[] ["EnFlo_Tunnel:Setpoint:Floor_Up_Y=-1585", "EnFlo_Tunnel:Setpoint:Floor_Up_Y=-1250", "EnFlo_Tunnel:Setpoint:Floor_Up_Y=-920", "EnFlo_Tunnel:Setpoint:Floor_Up_Y=-585", "EnFlo_Tunnel:Setpoint:Floor_Up_Y=-250", "EnFlo_Tunnel:Setpoint:Floor_Up_Y=80", "EnFlo_Tunnel:Setpoint:Floor_Up_Y=415", "EnFlo_Tunnel:Setpoint:Floor_Up_Y=750", "EnFlo_Tunnel:Setpoint:Floor_Up_Y=1080", "EnFlo_Tunnel:Setpoint:Floor_Up_Y=1415"] ("subarray")
        n176 = Array Size(array=w462) -> (size(s)=w461:i32)
        n177 = Array Size(array=w451) -> (size(s)=w450:i32)
        n178 = Array Size(array=w455) -> (size(s)=w460:i32)
        n179 = Array Subset(array=w459, index=w461, length=w460) -> (w457:dbl[])
        n180 = Build Array (concatenate)(w462, w455) -> (w463:string[])
        n181 = property on="Upstream Floor" class="XYGraph (strict)"("Active Plot"=w450, "Plot.Plot Name"="Setpoint") -> ()  [unwired: 2 in, 2 out]
        n182 = Bundle("Array"=dbl[] [-1585.0, -1250.0, -920.0, -585.0, -250.0, 80.0, 415.0, 750.0, 1080.0, 1415.0], w457) -> (w453:cluster{"Array":dbl[], dbl[]})  [unwired: 1 in]
        n183 = Build Array (concatenate)(w451, w453) -> (w452:cluster{"Array":dbl[], dbl[]}[])
      }
      frame "Upstream Floor Panel Powers" {
        w472 = string[] ["EnFlo_Tunnel:Power:Floor_Up_Y=-1585", "EnFlo_Tunnel:Power:Floor_Up_Y=-1250", "EnFlo_Tunnel:Power:Floor_Up_Y=-920", "EnFlo_Tunnel:Power:Floor_Up_Y=-585", "EnFlo_Tunnel:Power:Floor_Up_Y=-250", "EnFlo_Tunnel:Power:Floor_Up_Y=80", "EnFlo_Tunnel:Power:Floor_Up_Y=415", "EnFlo_Tunnel:Power:Floor_Up_Y=750", "EnFlo_Tunnel:Power:Floor_Up_Y=1080", "EnFlo_Tunnel:Power:Floor_Up_Y=1415"] ("subarray")
        n184 = Array Size(array=w479) -> (size(s)=w478:i32)
        n185 = Array Size(array=w468) -> (size(s)=w467:i32)
        n186 = Array Size(array=w472) -> (size(s)=w477:i32)
        n187 = Array Subset(array=w476, index=w478, length=w477) -> (w474:dbl[])
        n188 = Build Array (concatenate)(w479, w472) -> (w480:string[])
        n189 = property on="Upstream Floor" class="XYGraph (strict)"("Active Plot"=w467, "Plot.Plot Name"="Power") -> ()  [unwired: 2 in, 2 out]
        n190 = Bundle("Array"=dbl[] [-1585.0, -1250.0, -920.0, -585.0, -250.0, 80.0, 415.0, 750.0, 1080.0, 1415.0], w474) -> (w470:cluster{"Array":dbl[], dbl[]})  [unwired: 1 in]
        n191 = Build Array (concatenate)(w468, w470) -> (w469:cluster{"Array":dbl[], dbl[]}[])
      }
      frame "Upstream Above Floor Panel" {
        w489 = string[] ["EnFlo_Tunnel:Temp:Z=70_Y=-1585", "EnFlo_Tunnel:Temp:Z=70_Y=-1250", "EnFlo_Tunnel:Temp:Z=70_Y=-920", "EnFlo_Tunnel:Temp:Z=70_Y=-585", "EnFlo_Tunnel:Temp:Z=70_Y=-250", "EnFlo_Tunnel:Temp:Z=70_Y=80", "EnFlo_Tunnel:Temp:Z=70_Y=415", "EnFlo_Tunnel:Temp:Z=70_Y=750", "EnFlo_Tunnel:Temp:Z=70_Y=1080", "EnFlo_Tunnel:Temp:Z=70_Y=1415"] ("subarray")
        n192 = Array Size(array=w496) -> (size(s)=w495:i32)
        n193 = Array Size(array=w485) -> (size(s)=w484:i32)
        n194 = Array Size(array=w489) -> (size(s)=w494:i32)
        n195 = Array Subset(array=w493, index=w495, length=w494) -> (w491:dbl[])
        n196 = Build Array (concatenate)(w496, w489) -> (w497:string[])
        n197 = property on="Upstream Floor" class="XYGraph (strict)"("Active Plot"=w484, "Plot.Plot Name"="Z=70") -> ()  [unwired: 2 in, 2 out]
        n198 = Bundle("Array"=dbl[] [-1585.0, -1250.0, -920.0, -585.0, -250.0, 80.0, 415.0, 750.0, 1080.0, 1415.0], w491) -> (w487:cluster{"Array":dbl[], dbl[]})  [unwired: 1 in]
        n199 = Build Array (concatenate)(w485, w487) -> (w486:cluster{"Array":dbl[], dbl[]}[])
      }
      frame "Lab Stratification" {
        w516 = dbl[] [0.0, 6.0]
        w519 = 8 ("length")
        w531 = dbl[] [5.75, 4.5, 3.5, 2.5, 1.5, 0.5, 0.1, 0.0]
        n200 = Array Size(array=w534) -> (size(s)=w518:i32)
        n201 = Add(x=w518, y=w519) -> (x+y=w517:i32)
        n202 = Array Subset(array=w521, index=w517) -> (w520:dbl[])  [unwired: 1 in]
        n203 = Index Array(array=w520) -> (element #1=→"Delta T":dbl, element #2=w513:dbl, element #3=→"Heat Extraction kW":dbl, element #4=w515:dbl)  [unwired: 4 in]
        "Av Pre Inlet Temp" <- w513
        "Des Air Temp" <- w515
        n204 = Array Subset(array=w521, index=w518, length=w519) -> (w524:dbl[])
        n205 = for {
          N: 15 -> [_]
          tunnel: 2.43 -> [w542]
          tunnel: [w540] -> w528 mode=indexing
          i -> [w544]
          n206 = Multiply(x=0.1, y=w544) -> (x*y=w541:dbl)
          n207 = Subtract(x=w542, y=w541) -> (x-y=w540:dbl)
        }
        n208 = call <vilib>:"Interpolate 1D.vi"("xi"=w528, "X"=w531, "Y"=w524) -> ("yi"=w527:dbl[])  [unwired: 3 in, 5 out]
        n209 = Build Array(w515, w515) -> (w514:dbl[])
        n210 = Build Array(w513, w513) -> (w512:dbl[])
        n211 = local read "Heaters Enabled"() -> (w503:bool)
        n212 = Bundle(w524, w531) -> (w511:cluster{dbl[], dbl[]})  [unwired: 1 in]
        n213 = Bundle(w514, w516) -> (w510:cluster{dbl[], dbl[]})  [unwired: 1 in]
        n214 = Bundle(w512, w516) -> (w509:cluster{dbl[], dbl[]})  [unwired: 1 in]
        n215 = Bundle("yi"=w527, w507) -> (w526:cluster{"yi":dbl[], dbl[]})  [unwired: 1 in]
        n216 = case shown="False" w503 {
          tunnel: ["Get Server Values" "Inlet Heater Setpoint Values"] -> w502
          frame False {
          }
          frame True {
          }
        }
        n217 = Build Array(w511, w510, w509) -> (w508:cluster{dbl[], dbl[]}[])
        n218 = Build Array (concatenate)(w534, string[] ["EnFlo Lab:labstrat1:Z=5.75m Roof", "EnFlo Lab:labstrat1:Z=4.5m", "EnFlo Lab:labstrat1:Z=3.5m", "EnFlo Lab:labstrat1:Z=2.5m", "EnFlo Lab:labstrat1:Z=1.5m", "EnFlo Lab:labstrat1:Z=0.5m", "EnFlo Lab:labstrat1:Z=0.1m", "EnFlo Lab:labstrat1:Z=0m Floor", "EnFlo Lab:labstrat1:Delta T", "EnFlo_Tunnel:Temp:Pre_Inlet_Average", "EnFlo Lab:Heat:Extraction", "EnFlo Lab:Desired:Air Temp"] ("subarray")) -> (w535:string[])
        n219 = local read "Loop number"() -> (w501:i32)
        n220 = case shown="1, Default" w501 {
          tunnel: w508 -> [_ w537]
          frame 0 {
          }
          frame 1, Default {
            "Strat" <- w537
          }
        }
        n221 = Array Size(array=w504) -> (size(s)=w505:i32)
        n222 = Build Array (concatenate)(w504, w526) -> (w525:cluster{"yi":dbl[], dbl[]}[])
        n223 = property on="Inlet Heaters" class="XYGraph (strict)"("Active Plot"=w505, "Plot.Plot Name"="Lab Strat") -> ()  [unwired: 2 in, 2 out]
      }
      frame "Inlet Heater Setpoint Values" {
        w546 = string[] ["EnFlo_Tunnel:Setpoint:Inlet_Y=0_Z=1450", "EnFlo_Tunnel:Setpoint:Inlet_Y=0_Z=1350", "EnFlo_Tunnel:Setpoint:Inlet_Y=0_Z=1250", "EnFlo_Tunnel:Setpoint:Inlet_Y=0_Z=1150", "EnFlo_Tunnel:Setpoint:Inlet_Y=0_Z=1050", "EnFlo_Tunnel:Setpoint:Inlet_Y=0_Z=950", "EnFlo_Tunnel:Setpoint:Inlet_Y=0_Z=850", "EnFlo_Tunnel:Setpoint:Inlet_Y=0_Z=750", "EnFlo_Tunnel:Setpoint:Inlet_Y=0_Z=650", "EnFlo_Tunnel:Setpoint:Inlet_Y=0_Z=550", "EnFlo_Tunnel:Setpoint:Inlet_Y=0_Z=450", "EnFlo_Tunnel:Setpoint:Inlet_Y=0_Z=350", "EnFlo_Tunnel:Setpoint:Inlet_Y=0_Z=250", "EnFlo_Tunnel:Setpoint:Inlet_Y=0_Z=150", "EnFlo_Tunnel:Setpoint:Inlet_Y=0_Z=50"] ("subarray")
        n224 = Array Size(array=w561) -> (size(s)=w560:i32)
        n225 = Array Size(array=w549) -> (size(s)=w547:i32)
        n226 = property on="Inlet Heaters" class="XYGraph (strict)"("Active Plot"=w547, "Plot.Plot Name"="Inlet Setpoints") -> ()  [unwired: 2 in, 2 out]
        n227 = Array Size(array=w546) -> (size(s)=w559:i32)
        n228 = Array Subset(array=w558, index=w560, length=w559) -> (w551:dbl[])
        n229 = Bundle(w551, w550) -> (w557:cluster{dbl[], dbl[]})  [unwired: 1 in]
        n230 = for {
          tunnel: i32[] [14, 10, 5, 0] -> [w566] mode=indexing
          tunnel: w551 -> [w564]
          tunnel: [w565] -> w553 mode=indexing
          n231 = Index Array(array=w564, index=w566) -> (element=w565:dbl)
        }
        "Setpoints" <- w553
        n232 = Build Array (concatenate)(w561, w546) -> (w562:string[])
        n233 = Build Array (concatenate)(w549, w557) -> (w556:cluster{"yi":dbl[], dbl[]}[])
      }
      frame "Inlet Heater Power Values" {
        w568 = string[] ["EnFlo_Tunnel:Power:Inlet_Y=0_Z=1450", "EnFlo_Tunnel:Power:Inlet_Y=0_Z=1350", "EnFlo_Tunnel:Power:Inlet_Y=0_Z=1250", "EnFlo_Tunnel:Power:Inlet_Y=0_Z=1150", "EnFlo_Tunnel:Power:Inlet_Y=0_Z=1050", "EnFlo_Tunnel:Power:Inlet_Y=0_Z=950", "EnFlo_Tunnel:Power:Inlet_Y=0_Z=850", "EnFlo_Tunnel:Power:Inlet_Y=0_Z=750", "EnFlo_Tunnel:Power:Inlet_Y=0_Z=650", "EnFlo_Tunnel:Power:Inlet_Y=0_Z=550", "EnFlo_Tunnel:Power:Inlet_Y=0_Z=450", "EnFlo_Tunnel:Power:Inlet_Y=0_Z=350", "EnFlo_Tunnel:Power:Inlet_Y=0_Z=250", "EnFlo_Tunnel:Power:Inlet_Y=0_Z=150", "EnFlo_Tunnel:Power:Inlet_Y=0_Z=50"] ("subarray")
        n234 = Array Size(array=w581) -> (size(s)=w580:i32)
        n235 = Array Size(array=w570) -> (size(s)=w571:i32)
        n236 = Array Size(array=w568) -> (size(s)=w579:i32)
        n237 = Array Subset(array=w578, index=w580, length=w579) -> (w577:dbl[])
        n238 = Bundle(w577, w575) -> (w573:cluster{dbl[], dbl[]})  [unwired: 1 in]
        n239 = Build Array (concatenate)(w581, w568) -> (w582:string[])
        n240 = property on="Inlet Heaters" class="XYGraph (strict)"("Active Plot"=w571, "Plot.Plot Name"="Inlet Powers") -> ()  [unwired: 2 in, 2 out]
        n241 = Build Array (concatenate)(w570, w573) -> (w574:cluster{"yi":dbl[], dbl[]}[])
      }
      frame "Get Server Values" {
        n242 = local read "Loop number"() -> (w585:i32)
        n243 = Increment(x=w585) -> (x+1=w589:i32)
        n244 = local write "Loop number"(w589) -> ()
        n245 = case shown="Default" w585 {
          tunnel: w588 -> [_ w603 _]
          tunnel: [TRUE ("Top Level") w601 w636] -> w591
          frame 0 {
          }
          frame 1 {
            n246 = global read "Constants_global.vi" "Data Folder Local"() -> (w602:path)
            n247 = stacked-sequence {
              tunnel: w603 -> [w612 _]
              tunnel: w602 -> [w606 w629]
              tunnel: [w604 _] -> w601
              frame #0 {
                n248 = for {
                  tunnel: T2 {"Template Channel Name"="", "Description"="", "Tolerance"=0.0, "Precision"="", "Folder level"="", "Source"=[], "Replace"=[], "Summarise"=FALSE, "Dispose"=FALSE, "Min Value"="", "Maths"="", "Omit Rows Containing"=[], "Ignore When"=[], "Max Value"=""} ("Cluster") -> [w622]
                  tunnel: w612 -> [w615] mode=indexing
                  tunnel: [w621] -> w611 mode=indexing if=w617
                  shift-right: [w619] -> _
                  shift-left: string[] [] -> [w620]
                  tunnel: "Do not prompt me if this channnel is not found" -> [w614]
                  n249 = Search 1D Array(1D array=w620, element=w615) -> (index of element=w618:i32)  [unwired: 1 in]
                  n250 = Build Array(w615, w614) -> (w616:string[])
                  n251 = Bundle By Name(cluster=w622, "Template Channel Name"=w615, "Source"=w616) -> (w621:T2)
                  n252 = case shown="-1" w618 {
                    tunnel: w620 -> [w624 w628]
                    tunnel: [w624 w627] -> w619
                    tunnel: w615 -> [_ w626]
                    tunnel: [FALSE TRUE] -> w617
                    frame Default {
                    }
                    frame -1 {
                      n253 = Build Array (concatenate)(w628, w626) -> (w627:string[])
                    }
                  }
                }
                n254 = Build Path(base path=w606, name or relative path="EnFlo_Tunnel_Display_Template.xls") -> (appended path=w607:path)
                n255 = local read "Top Level"() -> (w604:bool)
                n256 = call "Read_Write_Temp_Cluster.vi"("Template Info Array"=w611, "Mode"=Global_mode."Write Global to File", "Template File"=w607) -> ()  [unwired: 2 in, 1 out]
              }
              frame #1 {
                n257 = Path To String(path=w629) -> (string=w630:string)
                n258 = call "Read_Write_Template.vi"("Mode"=Global_mode."Write Global to File", "Single Value In"=w630, "Data type"="Log Folder Name" ("Variable name")) -> ()  [unwired: 5 in, 8 out]
              }
            }
          }
          frame Default {
            n259 = global read "Results_plotter_Global.vi" "Plot EnFlo Tunnel Display"() -> (w635:bool)
            n260 = Or(x=w635, y="Stop Button") -> (x .or. y?=w633:bool)
            n261 = Not(x=w633) -> (.not. x?=w636:bool)
          }
        }
        n262 = Multiply(x="History in Minutes", y=60.0) -> (x*y=w594:dbl)
        n263 = call "Get_Channel_averages.vi"("Desired Ch Names"=w588, "Averaging time (mins)"="Averaging time (mins)", "End Offset Sec (0)"=w594) -> ("number"=w590:dbl[])  [unwired: 2 out]
        n264 = case shown="1, Default" w585 {
          tunnel: w587 -> [_ w599]
          tunnel: w586 -> [_ w598]
          tunnel: w584 -> [_ w597]
          frame 0 {
          }
          frame 1, Default {
            "Inlet Heaters" <- w598
            "Panel Temps" <- w599
            "Upstream Floor" <- w597
          }
        }
      }
    }
  }
